vi "climb.vi"(0 "Setpoint ARM":dbl, 1 "Operation":T1=enum."Read Current", 2 "Reset":bool, 3 "Description":string, 4 "Defense mode?":bool, 5 "Roll":dbl, 7 "Enum":enum16{"Level 1-3", "Level 1-2", "Level 2-3"}(ring), 9 "Setpoint WHEELS":dbl, 11 "Command Info In":T2, 12 "Pitch":dbl, 13 "New Pos?":bool, 14 "Speedy Tilt":cluster{"Right":bool, "Left":bool}={"Right"=TRUE, "Left"=TRUE}) -> (15 "Command Info Out":T2)   [LabVIEW 2018]
doc: "This template is useful for immediate subsystem actions that do not need deadband filtering\n\nBe sure to right-click and select New from Template and save with a new command name."
uses:
  <vilib>/Rock Robotics/WPI/Framework/Command Status Info.ctl
  <vilib>/Rock Robotics/WPI/Framework/Completion Status.ctl
  <vilib>/Rock Robotics/WPI/Framework/Completion Notifier.ctl
  Implementation/Climb Operations.ctl
  Implementation/Climb Setpoints.ctl
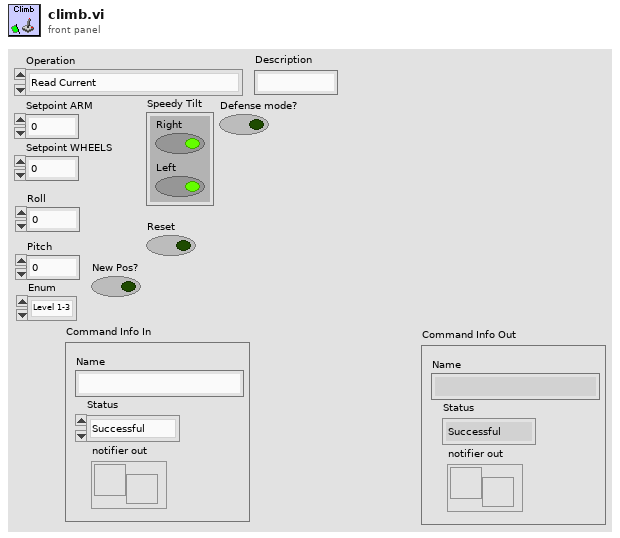
[diagram p1: front panel]
types:
  T1 = typedef "Climb Operations.ctl" = enum16{"Reserve", "Read Current", "Immediate", "Ready", "Auto-Climb", "Reset/Turbo-Tilt", "Manual Climb"}
  T2 = typedef "Command Status Info.ctl" = cluster{"Name":string, "Status":T3, "notifier out":T4}
  T3 = typedef "Completion Status.ctl" = enum16{"Successful", "Aborted", "Incomplete"}
  T4 = typedef "Completion Notifier.ctl" = refnum<notifier>
  T5 = typedef "Climb Setpoints.ctl" = cluster{"Operation":T1, "Setpoint Rhino":dbl, "Setpoint WHEELS":dbl, "Roll":dbl, "Pitch":dbl, "Reset":bool, "Speedy Tilt":cluster{"Right":bool, "Left":bool}, "Climb":enum16{"Level 1-3", "Level 1-2", "Level 2-3"}, "New Pos?":bool, "Defense mode?":bool}
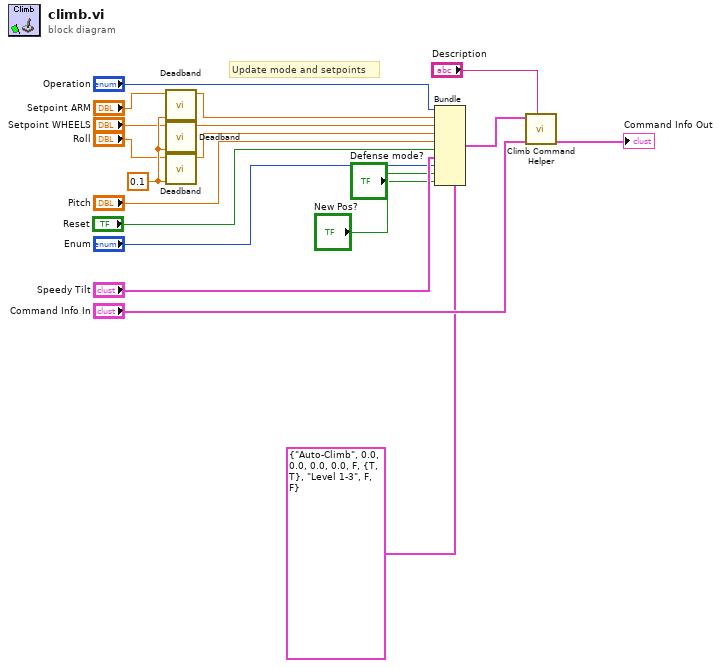
[diagram p0: block diagram]
diagram:
  w14 = 0.1 ("Deadband")
  # "Update mode and setpoints"
  n1 = call "Deadband.vi"("Deadband"=w14, "Input"="Setpoint ARM") -> ("f"=w9:dbl)  [unwired: 9 in]
  n2 = call "Deadband.vi"("Deadband"=w14, "Input"="Setpoint WHEELS") -> ("f"=w8:dbl)  [unwired: 9 in]
  n3 = call "Deadband.vi"("Deadband"=w14, "Input"="Roll") -> ("f"=w10:dbl)  [unwired: 9 in]
  n4 = Bundle(cluster=T5 {"Operation"=enum."Auto-Climb", "Setpoint Rhino"=0.0, "Setpoint WHEELS"=0.0, "Roll"=0.0, "Pitch"=0.0, "Reset"=FALSE, "Speedy Tilt"={"Right"=TRUE, "Left"=TRUE}, "Climb"=enum."Level 1-3", "New Pos?"=FALSE, "Defense mode?"=FALSE} ("SubSystem Data"), "Operation"="Operation", "Setpoint Rhino"=w9, "Setpoint WHEELS"=w8, "Roll"=w10, "Pitch"="Pitch", "Reset"="Reset", "Speedy Tilt"="Speedy Tilt", "Climb"="Enum", "New Pos?"="New Pos?", "Defense mode?"="Defense mode?") -> (w15:T5)
  n5 = call "Climb Command Helper.vi"("Description"="Description", "Command Info In"="Command Info In", "SubSystem Data"=w15) -> ("Command Info Out"=→"Command Info Out":T2)  [unwired: 6 in, 2 out]
